vi "_ReadCommand.vi"(7 "Disable MAV check (F)":bool, 8 "error in":errorcluster, 11 "Instrument Channel":string="GPIB/0:4,0") -> (0 "error out":errorcluster, 2 "Response":string, 3 "Instrument Channel out":string="GPIB/0:4,0")   [LabVIEW 2010]
doc: "Reads string from instrument channel."
panel:
  out "byte count":u32
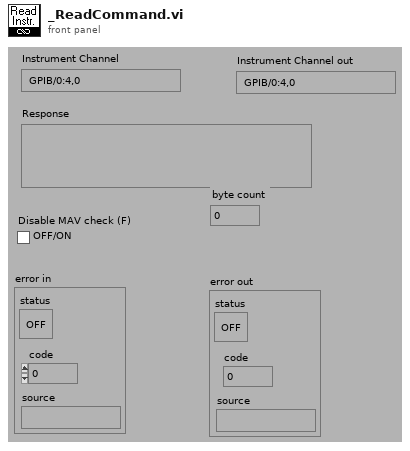
[diagram p1: front panel]
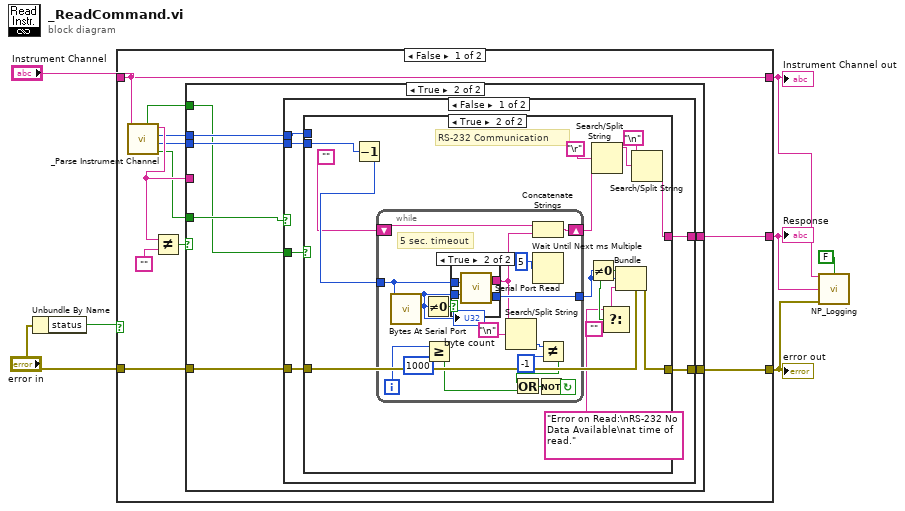
[diagram p0: block diagram]
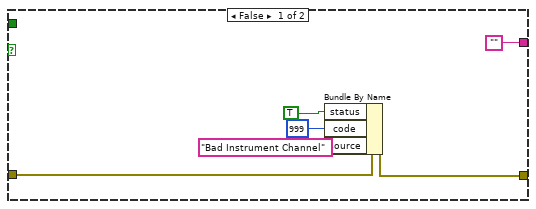
[diagram p2: hidden frame]
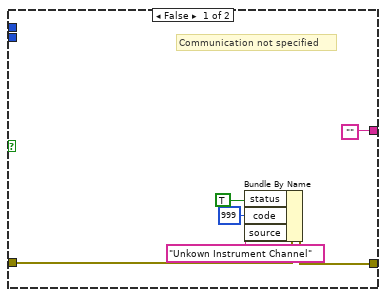
[diagram p3: hidden frame]
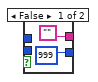
[diagram p4: hidden frame]
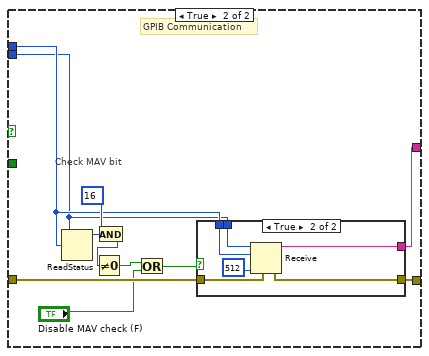
[diagram p5: hidden frame]
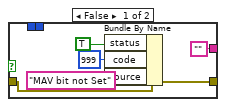
[diagram p6: hidden frame]
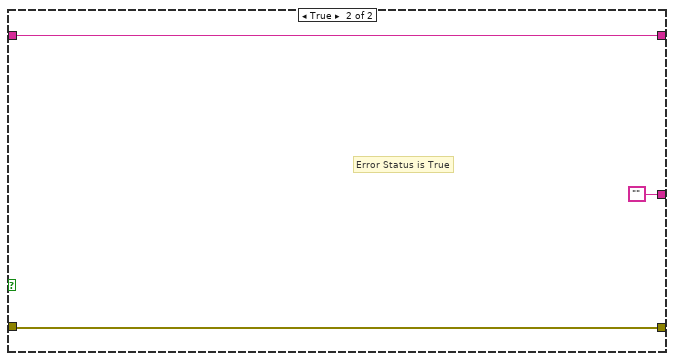
[diagram p7: hidden frame]
diagram:
  n1 = Unbundle By Name("error in") -> ("status"=w6:bool)
  n2 = case shown="False" w6 {
    tunnel: "error in" -> [w18 w106]
    tunnel: "Instrument Channel" -> [w14 w107]
    tunnel: [w14 w107] -> w4
    tunnel: [w13 ""] -> w1
    tunnel: [w12 w106] -> w3
    frame False {
      n3 = call <userlib>:"_Parse Instrument Channel.vi"("Instrument Channel"=w14) -> ("T - GPIB, F - RS232"=w11:bool, "Hardware Address"=w9:i32, "Instrument Address"=w10:i16, "Instrument Channel out"=w15:string, "Valid String"=w8:bool)  [unwired: 6 in]
      n4 = Not Equal?(x=w15, y="") -> (x != y?=w16:bool)
      n5 = case shown="True" w16 {
        tunnel: w18 -> [w21 w31]
        tunnel: [w20 w30] -> w12
        tunnel: w15 -> [_ _]
        tunnel: ["" w29] -> w13
        tunnel: w11 -> [_ w28]
        tunnel: w10 -> [_ w27]
        tunnel: w9 -> [_ w26]
        tunnel: w8 -> [_ w25]
        frame False {
          n6 = Bundle By Name(cluster=w21, "status"=TRUE, "code"=999, "source"="Bad Instrument Channel") -> (w20:errorcluster)
        }
        frame True {
          n7 = case shown="False" w28 {
            tunnel: w31 -> [w37 w92]
            tunnel: [w36 w91] -> w30
            tunnel: [w35 w90] -> w29
            tunnel: w27 -> [w34 w83]
            tunnel: w26 -> [w32 w82]
            tunnel: w25 -> [w33 _]
            frame False {
              n8 = case shown="True" w33 {
                tunnel: w37 -> [w39 w55]
                tunnel: [w38 w56] -> w36
                tunnel: ["" w48] -> w35
                tunnel: w34 -> [_ _]
                tunnel: w32 -> [_ w44]
                frame False {
                  # "Communication not specified"
                  n9 = Bundle By Name(cluster=w39, "status"=TRUE, "code"=999, "source"="Unkown Instrument Channel") -> (w38:errorcluster)
                }
                frame True {
                  # "RS-232 Communication"
                  n10 = Decrement(x=w44) -> (x-1=w47:i32)
                  n11 = while {
                    shift-left: "" -> [w70]
                    shift-right: [w71] -> w45
                    tunnel: w47 -> [w74]
                    tunnel: [w75] -> w54
                    i -> [w65]
                    stop <- w59 continue-if-true
                    # "5 sec. timeout"
                    n12 = call <vilib>:"Bytes At Serial Port.vi"("port number"=w74) -> ("byte count"=w73:u32)  [unwired: 1 out]
                    "byte count" <- w73
                    n13 = Not Equal To 0?(x=w73) -> (x != 0?=w72:bool)
                    n14 = Greater Or Equal?(x=w65, y=1000) -> (x >= y?=w60:bool)
                    n15 = case shown="True" w72 {
                      tunnel: ["" w81] -> w68
                      tunnel: w74 -> [_ w80]
                      tunnel: w73 -> [_ w79]
                      tunnel: [999 w78] -> w75
                      frame False {
                      }
                      frame True {
                        n16 = call <vilib>:"Serial Port Read.vi"("requested byte count"=w79, "port number"=w80) -> ("error code"=w78:i32, "string read"=w81:string)
                      }
                    }
                    n17 = Search/Split String(string=w68, search string/char (-)="\n") -> (offset of match=w67:i32)  [unwired: 1 in, 2 out]
                    n18 = Concatenate Strings(w70, w68) -> (w71:string)
                    n19 = Wait Until Next ms Multiple(millisecond multiple=5) -> ()  [unwired: 1 out]
                    n20 = Not Equal?(x=w67, y=-1) -> (x != y?=w61:bool)
                    n21 = Or(x=w61, y=w60) -> (x .or. y?=w62:bool)
                    n22 = Not(x=w62) -> (.not. x?=w59:bool)
                  }
                  n23 = Not Equal To 0?(x=w54) -> (x != 0?=w58:bool)
                  n24 = Search/Split String(string=w45, search string/char (-)="\r") -> (substring before match=w49:string)  [unwired: 1 in, 2 out]
                  n25 = Select(t="Error on Read:\nRS-232 No Data Available\nat time of read.", s=w58, f="") -> (s? t:f=w57:string)
                  n26 = Bundle(cluster=w55, "status"=w58, "code"=w54, "source"=w57) -> (w56:errorcluster)
                  n27 = Search/Split String(string=w49, search string/char (-)="\n") -> (substring before match=w48:string)  [unwired: 1 in, 2 out]
                }
              }
            }
            frame True {
              # "Check MAV bit"
              # "GPIB Communication"
              n28 = ReadStatus(4:w83, 5:w82) -> (2:w89:i16)  [unwired: 1 in, 2 out]
              n29 = And(x=u16 16, y=w89) -> (x .and. y?=w86:u16)
              n30 = Not Equal To 0?(x=w86) -> (x != 0?=w87:bool)
              n31 = Or(x=w87, y="Disable MAV check (F)") -> (x .or. y?=w85:bool)
              n32 = case shown="True" w85 {
                tunnel: ["" w104] -> w90
                tunnel: [w93 w102] -> w91
                tunnel: w92 -> [w94 w101]
                tunnel: w83 -> [_ w100]
                tunnel: w82 -> [_ w99]
                frame False {
                  n33 = Bundle By Name(cluster=w94, "status"=TRUE, "code"=999, "source"="MAV bit not Set") -> (w93:errorcluster)
                }
                frame True {
                  n34 = Receive(4:w101, 6:512, 8:w100, 9:w99) -> (0:w102:errorcluster, 3:w104:string)  [unwired: 1 in, 2 out]
                }
              }
            }
          }
        }
      }
    }
    frame True {
      # "Error Status is True"
    }
  }
  "Instrument Channel out" <- w4
  "error out" <- w3
  "Response" <- w1
  n35 = call <userlib>:"NP_Logging.vi"("Instrument Channel"=w4, "String 1 Enable (T)"=FALSE, "String 2 {Read} (in)"=w1, "error in (no error)"=w3) -> ()  [unwired: 8 in, 4 out]
